vi "Memory.Pointer.Write.Safe.1D.DBL.vi"(8 "error in (no error)":errorcluster, 9 "count":u64 format="%d elements", 10 "buffer in":dbl[](array[numeric]), 11 "pointer in":refnum<class "Memory.Pointer.lvclass">) -> (0 "error out":errorcluster, 2 "buffer out":dbl[](array[numeric]), 3 "pointer out":refnum<class "Memory.Pointer.lvclass">)   [LabVIEW 2016, in "Memory Manager.lvlib" / "Memory.Pointer.lvclass"]
doc: "Writes <b>count</b> elements from the provided <b>buffer</b> to the address specified by <b>pointer</b>.\n\n<b>Note:</b> This VI is <b>safe</b>.\n\nSafe means that this function evaluates the size parameter of <b>pointer</b> to ensure that is inbounds of allocated memory before peforming a memory read/write. Reading/writing more data to a pointer than it has allocated can corrupt or crash LabVIEW."
uses:
  Memory.Pointer.lvclass
  Memory.Pointer.lvclass/Memory.Pointer.ctl
  Accessors/Get Address.vi
panel:
  out "count out":u64 format="%d elements"
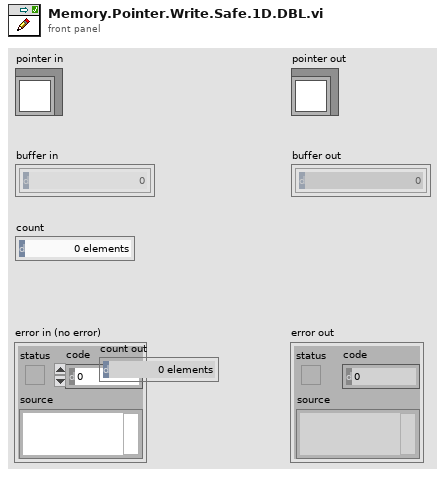
[diagram p1: front panel]
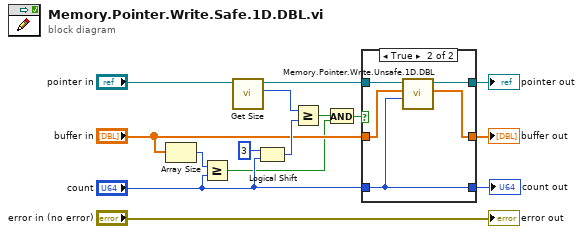
[diagram p0: block diagram]
diagram:
  n1 = Array Size(array="buffer in") -> (size(s)=w5:i32)
  n2 = Greater Or Equal?(x=w5, y="count") -> (x >= y?=w1:bool)
  n3 = call "Get Size.vi"("Pointer in"="pointer in") -> ("size"=w13:u64, "Pointer out"=w11:refnum<class "Memory.Pointer.lvclass">)  [unwired: 8 in, 1 out]
  n4 = Logical Shift(y=i16 3, x="count") -> (x << y=w12:u64)
  n5 = Greater Or Equal?(x=w13, y=w12) -> (x >= y?=w2:bool)
  n6 = And(x=w2, y=w1) -> (x .and. y?=w3:bool)
  n7 = case shown="True" w3 {
    tunnel: w11 -> [w16 w23]
    tunnel: [w16 w22] -> w10
    tunnel: "buffer in" -> [w17 w21]
    tunnel: "count" -> [w18 w19]
    tunnel: [w17 w20] -> w9
    tunnel: [w18 w19] -> w7
    frame False {
    }
    frame True {
      n8 = call "Memory.Pointer.Write.Unsafe.1D.DBL.vi"("count"=w19, "buffer in"=w21, "pointer in"=w23) -> ("buffer out"=w20:dbl[], "pointer out"=w22:refnum<class "Memory.Pointer.lvclass">)  [unwired: 6 in, 1 out]
    }
  }
  "pointer out" <- w10
  "buffer out" <- w9
  "count out" <- w7
  "error out" <- "error in (no error)"
